vi "GetTaggedPhotons.vi"(7 "screen status":T3, 8 "fft cluster":T4, 9 "FFT reference":refnum<vi>, 10 "unit":T2, 11 "I (current unit)":dbl[][](array[numeric])) -> (3 "output cluster 2":T1)   [LabVIEW 2018, in "Photon Filtering.lvlib"]
uses:
  Photon Filtering.lvlib
  Ximea programs/typedef/ImageUnit.ctl
  OutputPhotonCluster.ctl
  <vilib>/Analysis/2dsp.llb/2D Complex FFT.vi
  <vilib>/Analysis/2dsp.llb/2D Inverse Complex FFT.vi
  Ximea programs/References.vi
  <vilib>/Analysis/NI_AALPro.lvlib
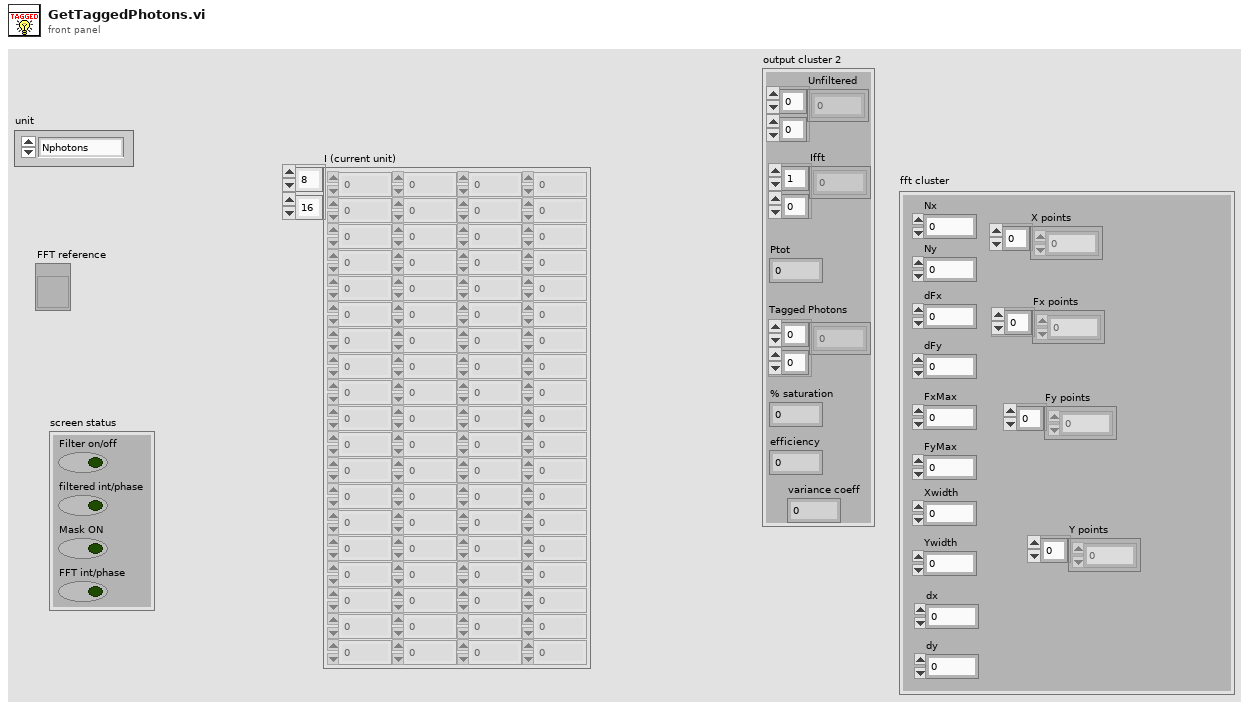
[diagram p1: front panel]
types:
  T1 = typedef "Photon Filtering.lvlib/OutputPhotonCluster.ctl" = cluster{"Unfiltered":dbl[][], "Ifft":dbl[][], "Ptot":dbl, "Tagged Photons":dbl[][], "% saturation":dbl, "efficiency":dbl, "variance coeff":dbl}
  T2 = typedef "ImageUnit.ctl" = enum16{"Nphotons", "Efficiency", "I(uW/cm^2)", "I(nW/cm^2)", "Nelectrons", "I[W/cm^2]", "counts"}
  T3 = cluster{"Filter on/off":bool, "filtered int/phase":bool, "Mask ON":bool, "FFT int/phase":bool}
  T4 = cluster{"dFx":dbl, "dFy":dbl, "Nx":i32, "Ny":i32, "FxMax":dbl, "FyMax":dbl, "Xwidth":dbl, "Ywidth":dbl, "dx":dbl, "dy":dbl, "Fx points":dbl[], "X points":dbl[], "Y points":dbl[], "Fy points":dbl[]}
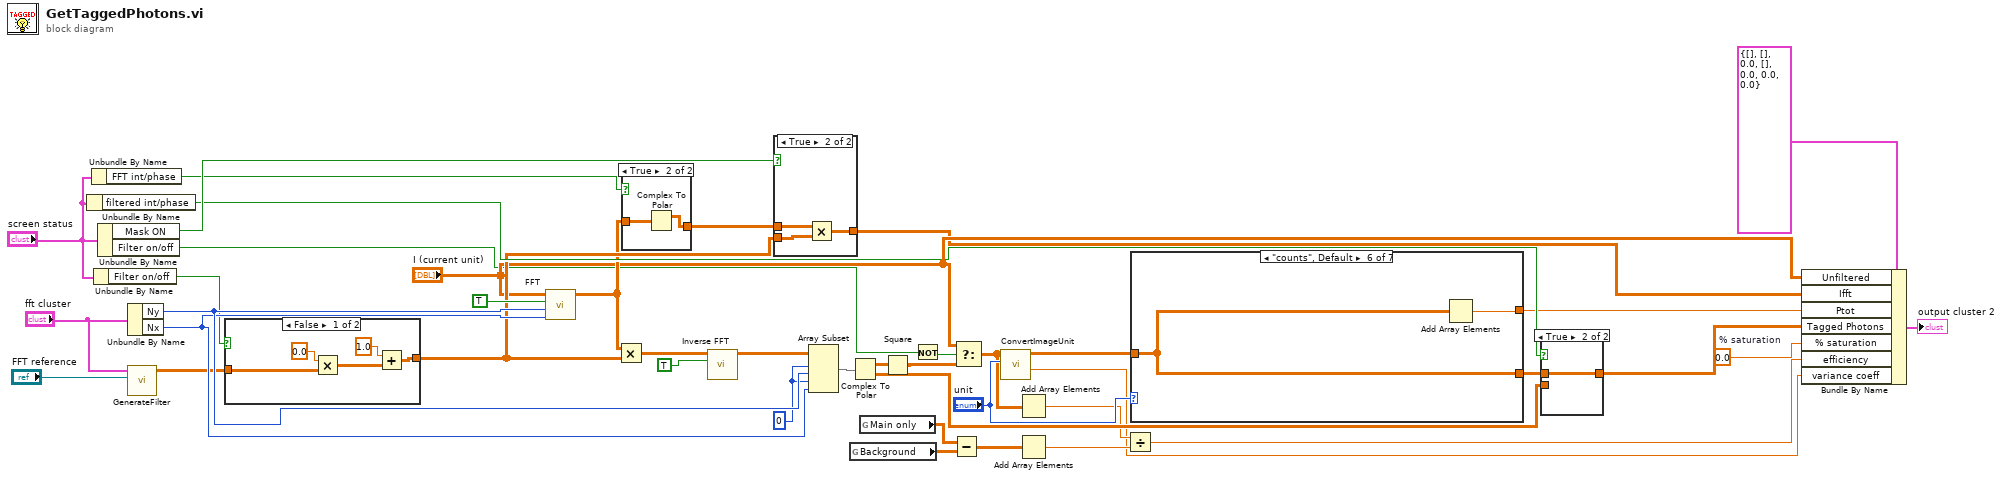
[diagram p0: block diagram]
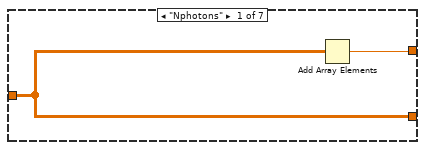
[diagram p2: hidden frame]
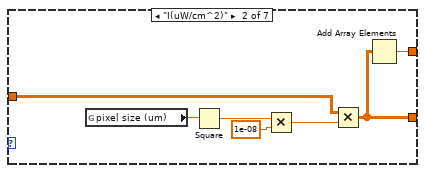
[diagram p3: hidden frame]
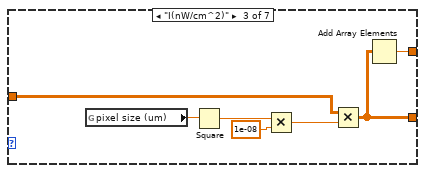
[diagram p4: hidden frame]
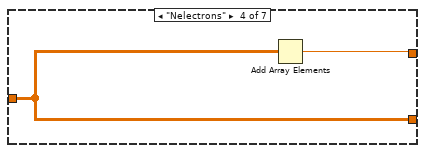
[diagram p5: hidden frame]
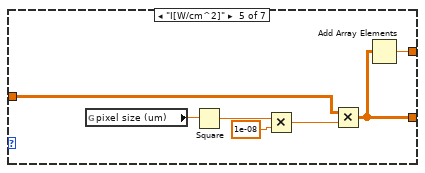
[diagram p6: hidden frame]
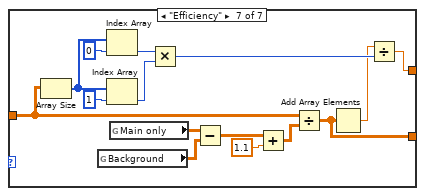
[diagram p7: hidden frame]
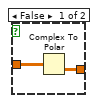
[diagram p8: hidden frame]
diagram:
  w9 = 0.0  # % saturation
  w15 = 0 ("index")
  n1 = Unbundle By Name("screen status") -> ("filtered int/phase"=w35:bool)
  n2 = Unbundle By Name("screen status") -> ("FFT int/phase"=w32:bool)
  n3 = Unbundle By Name("screen status") -> ("Filter on/off"=w37:bool)
  n4 = Unbundle By Name("screen status") -> ("Mask ON"=w36:bool, "Filter on/off"=w4:bool)
  n5 = Unbundle By Name("fft cluster") -> ("Ny"=w39:i32, "Nx"=w38:i32)
  n6 = call "GenerateFilter.vi"("FFT reference"="FFT reference", "FFT cluster IN"="fft cluster") -> ("filter out"=w28:dbl[][])  [unwired: 9 in]
  n7 = case shown="False" w37 {
    tunnel: [w44 w48] -> w30
    tunnel: w28 -> [w43 w48]
    frame False {
      n8 = Multiply(x=0.0, y=w43) -> (x*y=w45:dbl[][])
      n9 = Add(x=1.0, y=w45) -> (x+y=w44:dbl[][])
    }
    frame True {
    }
  }
  n10 = call-poly <vilib>:"FFT.vi"("n"=w38, "m"=w39, "shift?"=TRUE, "X"="I (current unit)") -> ("FFT {X}"=w27:cdb[][])  [unwired: 6 in, 1 out]
  n11 = Multiply(x=w27, y=w30) -> (x*y=w40:cdb[][])
  n12 = case shown="True" w32 {
    tunnel: [w49 w51] -> w34
    tunnel: w27 -> [w50 w52]
    frame False {
      n13 = Complex To Polar(r * e^(i*theta)=w50) -> (theta=w49:dbl[][])  [unwired: 1 out]
    }
    frame True {
      n14 = Complex To Polar(r * e^(i*theta)=w52) -> (r=w51:dbl[][])  [unwired: 1 out]
    }
  }
  n15 = call-poly <vilib>:"Inverse FFT.vi"("shift?"=TRUE, "FFT {x}"=w40) -> ("X"=w31:cdb[][])  [unwired: 8 in, 1 out]
  n16 = case shown="True" w36 {
    tunnel: [w53 w54] -> w5
    tunnel: w34 -> [w53 w55]
    tunnel: w30 -> [_ w56]
    frame False {
    }
    frame True {
      n17 = Multiply(x=w55, y=w56) -> (x*y=w54:dbl[][])
    }
  }
  n18 = Array Subset(array=w31, index (row)=w15, length (row)=w39, index (col)=w15, length (col)=w38) -> (w24:cdb[][])
  n19 = global read "References.vi" "Background"() -> (w20:dbl[][])
  n20 = Complex To Polar(r * e^(i*theta)=w24) -> (r=w2:dbl[][], theta=w26:dbl[][])
  n21 = global read "References.vi" "Main only"() -> (w21:dbl[][])
  n22 = Square(x=w2) -> (x^2=w1:dbl[][])
  n23 = Not(x=w4) -> (.not. x?=w3:bool)
  n24 = Subtract(x=w21, y=w20) -> (x-y=w19:dbl[][])
  n25 = Select(t="I (current unit)", s=w3, f=w1) -> (s? t:f=w14:dbl[][])
  n26 = call "ConvertImageUnit.vi"("unit"="unit", "Images in Counts"=w14) -> ("shot noise coefficient (sigma2)"=w11:dbl, "converted image"=w18:dbl[][])  [unwired: 8 in]
  n27 = Add Array Elements(numeric array=w14) -> (sum=w17:dbl)
  n28 = Add Array Elements(numeric array=w19) -> (sum=w16:dbl)
  n29 = Divide(x=w17, y=w16) -> (x/y=w8:dbl)
  n30 = case shown="\"counts\", Default" "unit" {
    tunnel: [w58 w59 w67 w74 w76 w83 w93] -> w23
    tunnel: w18 -> [w58 w61 w68 w74 w77 w83 w86]
    tunnel: [w57 w60 w66 w73 w75 w82 w84] -> w7
    frame "Nphotons" {
      n31 = Add Array Elements(numeric array=w58) -> (sum=w57:dbl)
    }
    frame "I(uW/cm^2)" {
      n32 = global read "References.vi" "pixel size (um)"() -> (w64:dbl)
      n33 = Square(x=w64) -> (x^2=w65:dbl)
      n34 = Multiply(x=w65, y=1e-08) -> (x*y=w62:dbl)
      n35 = Multiply(x=w61, y=w62) -> (x*y=w59:dbl[][])
      n36 = Add Array Elements(numeric array=w59) -> (sum=w60:dbl)
    }
    frame "I(nW/cm^2)" {
      n37 = global read "References.vi" "pixel size (um)"() -> (w71:dbl)
      n38 = Square(x=w71) -> (x^2=w72:dbl)
      n39 = Multiply(x=w72, y=1e-08) -> (x*y=w69:dbl)
      n40 = Multiply(x=w68, y=w69) -> (x*y=w67:dbl[][])
      n41 = Add Array Elements(numeric array=w67) -> (sum=w66:dbl)
    }
    frame "Nelectrons" {
      n42 = Add Array Elements(numeric array=w74) -> (sum=w73:dbl)
    }
    frame "I[W/cm^2]" {
      n43 = global read "References.vi" "pixel size (um)"() -> (w80:dbl)
      n44 = Square(x=w80) -> (x^2=w81:dbl)
      n45 = Multiply(x=w81, y=1e-08) -> (x*y=w78:dbl)
      n46 = Multiply(x=w77, y=w78) -> (x*y=w76:dbl[][])
      n47 = Add Array Elements(numeric array=w76) -> (sum=w75:dbl)
    }
    frame "counts", Default {
      n48 = Add Array Elements(numeric array=w83) -> (sum=w82:dbl)
    }
    frame "Efficiency" {
      n49 = Array Size(array=w86) -> (size(s)=w88:i32[])
      n50 = global read "References.vi" "Background"() -> (w95:dbl[][])
      n51 = Index Array(array=w88, index=0) -> (element=w90:i32)
      n52 = Index Array(array=w88, index=1) -> (element=w89:i32)
      n53 = global read "References.vi" "Main only"() -> (w96:dbl[][])
      n54 = Multiply(x=w90, y=w89) -> (x*y=w87:i32)
      n55 = Subtract(x=w96, y=w95) -> (x-y=w94:dbl[][])
      n56 = Add(x=w94, y=1.1 ("Numeric")) -> (x+y=w97:dbl[][])
      n57 = Divide(x=w86, y=w97) -> (x/y=w93:dbl[][])
      n58 = Add Array Elements(numeric array=w93) -> (sum=w85:dbl)
      n59 = Divide(x=w85, y=w87) -> (x/y=w84:dbl)
    }
  }
  n60 = case shown="True" w35 {
    tunnel: [w99 w100] -> w10
    tunnel: w26 -> [w99 _]
    tunnel: w23 -> [_ w100]
    frame False {
    }
    frame True {
    }
  }
  n61 = Bundle By Name(cluster=T1 {"Unfiltered"=[], "Ifft"=[], "Ptot"=0.0, "Tagged Photons"=[], "% saturation"=0.0, "efficiency"=0.0, "variance coeff"=0.0} ("output cluster"), "Unfiltered"="I (current unit)", "Ifft"=w5, "Ptot"=w7, "Tagged Photons"=w10, "% saturation"=w9, "efficiency"=w8, "variance coeff"=w11) -> (→"output cluster 2":T1)
